vi "commandManipulateM1M3.vi"(8 "error in (no error)":errorcluster, 10 "CommandManipulateM1M3 in":T1, 11 "M1M3SAL in":refnum<class "M1M3SAL.lvclass">) -> (0 "error out":errorcluster, 2 "CommandManipulateM1M3 out":T1, 3 "M1M3SAL out":refnum<class "M1M3SAL.lvclass">)   [LabVIEW 2016, in "M1M3SupportCommunicator.lvlib" / "M1M3SAL.lvclass"]
uses:
  M1M3SAL.lvclass
  DataTypes/Topics/CommandManipulateM1M3.ctl
  DataTypes/Topics/Parts/CommandId.ctl
  DataTypes/MessageHeader.ctl
  DataTypes/MessageTypes.ctl
  DataTypes/MessageTopics.ctl
  M1M3SAL.lvclass/M1M3SAL.ctl
  writeU8.vi
  writeI32.vi
  M1M3SupportCommunicator.lvlib
  DataTypes/Topics/M1M3SupportTopics.lvlib
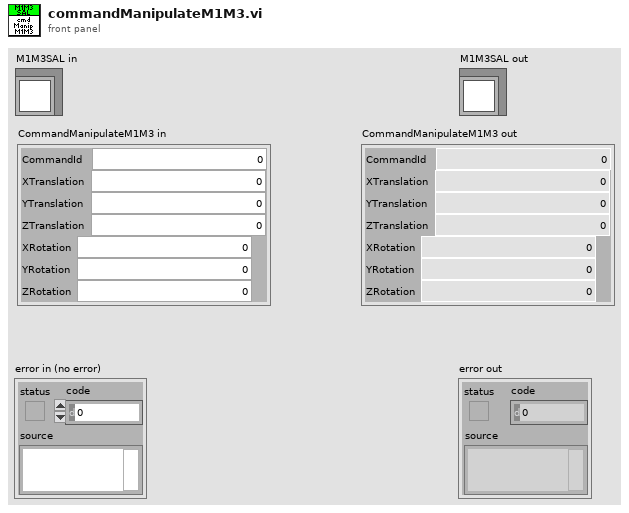
[diagram p1: front panel]
types:
  T1 = typedef "M1M3SupportTopics.lvlib/CommandManipulateM1M3.ctl" = cluster{"CommandId":T2, "XTranslation":dbl, "YTranslation":dbl, "ZTranslation":dbl, "XRotation":dbl, "YRotation":dbl, "ZRotation":dbl}
  T2 = typedef "M1M3SupportTopics.lvlib/CommandId.ctl" = i32
  T3 = typedef "M1M3SupportCommunicator.lvlib/MessageHeader.ctl" = cluster{"Type":T4, "Topic":T5, "Size":i32}
  T4 = typedef "M1M3SupportCommunicator.lvlib/MessageTypes.ctl" = enum8{"None", "PutSample", "GetNextSample", "LogEvent", "GetEvent", "IssueCommand", "CommandId", "WaitForCompletion", "AcceptCommand", "AckCommand"}
  T5 = typedef "M1M3SupportCommunicator.lvlib/MessageTopics.ctl" = enum8{"None", "ForceActuatorData", "MirrorForceData", "HardpointData", "AirData", "DynamicData", "FPGAData", "IMSData", "ForceActuatorStatus", "ElevationData", "HardpointStatus", "HardpointActuatorChase", "AirStatus", "ForceActuatorSafetyChecks", "ForceActuatorTest", "ActuatorBroadcastCounter", "StatusChecks", "CellChecks", "HardpointActuatorBreakaway", "RaiseMirrorComplete", "ILCCommunication", "ElevationAngleChecks", "DetailedState", "ServoLoops", "ForceActuatorInfo", "LowerMirrorComplete", "HardpointActuatorInfo", "SettingsApplied", "ErrorCode", "StartupChecks", "SummaryState", "SettingVersions", "ActuatorTestStatus", "AppliedSettingsMatchStart", "Enable", "EnterMaintenance", "Standby", "AbortLowerM1M3", "ApplyAberrationByForces", "ApplyAOSCorrectionByBendingModes", "ClearAOSCorrection", "Start", "RaiseM1M3", "TestForceActuator", "LowerM1M3", "ApplyAOSCorrectionByForces", "Disable", "ApplyAberationByBendingMode", "TestHardpoint", "ManipulateM1M3", "ClearAberration", "Exit", "TestAir", "AbortRaiseM1M3", "MoveHardpointActuators", "ExitMaintenance", "Shutdown"}
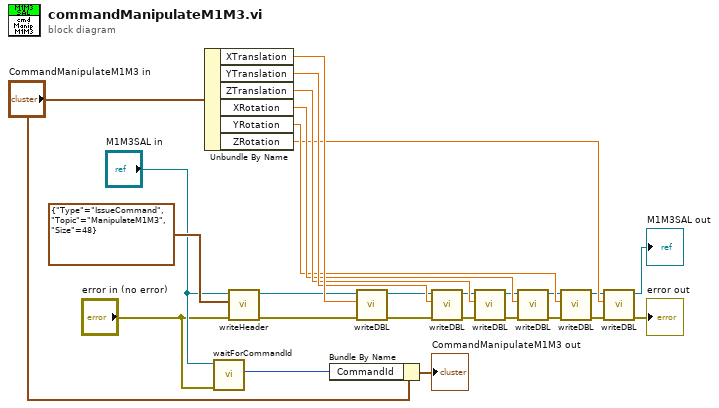
[diagram p0: block diagram]
diagram:
  n1 = Unbundle By Name("CommandManipulateM1M3 in") -> ("XTranslation"=w21:dbl, "YTranslation"=w20:dbl, "ZTranslation"=w19:dbl, "XRotation"=w18:dbl, "YRotation"=w17:dbl, "ZRotation"=w16:dbl)
  n2 = call "waitForCommandId.vi"("error in (no error)"="error in (no error)", "M1M3SAL in"="M1M3SAL in") -> ("CommandId"=w25:T2)  [unwired: 7 in, 2 out]
  n3 = call "writeHeader.vi"("error in (no error)"="error in (no error)", "MessageHeader"=T3 {"Type"=enum."IssueCommand", "Topic"=enum."ManipulateM1M3", "Size"=48}, "M1M3SAL in"="M1M3SAL in") -> ("error out"=w14:errorcluster, "M1M3SAL out"=w7:refnum<class "M1M3SAL.lvclass">)  [unwired: 7 in]
  n4 = Bundle By Name(cluster="CommandManipulateM1M3 in", "CommandId"=w25) -> (→"CommandManipulateM1M3 out":T1)
  n5 = call "writeDBL.vi"("error in (no error)"=w14, "Input"=w21, "M1M3SAL in"=w7) -> ("error out"=w13:errorcluster, "M1M3SAL out"=w6:refnum<class "M1M3SAL.lvclass">)  [unwired: 7 in]
  n6 = call "writeDBL.vi"("error in (no error)"=w13, "Input"=w20, "M1M3SAL in"=w6) -> ("error out"=w12:errorcluster, "M1M3SAL out"=w5:refnum<class "M1M3SAL.lvclass">)  [unwired: 7 in]
  n7 = call "writeDBL.vi"("error in (no error)"=w12, "Input"=w19, "M1M3SAL in"=w5) -> ("error out"=w11:errorcluster, "M1M3SAL out"=w4:refnum<class "M1M3SAL.lvclass">)  [unwired: 7 in]
  n8 = call "writeDBL.vi"("error in (no error)"=w11, "Input"=w18, "M1M3SAL in"=w4) -> ("error out"=w10:errorcluster, "M1M3SAL out"=w3:refnum<class "M1M3SAL.lvclass">)  [unwired: 7 in]
  n9 = call "writeDBL.vi"("error in (no error)"=w10, "Input"=w17, "M1M3SAL in"=w3) -> ("error out"=w9:errorcluster, "M1M3SAL out"=w2:refnum<class "M1M3SAL.lvclass">)  [unwired: 7 in]
  n10 = call "writeDBL.vi"("error in (no error)"=w9, "Input"=w16, "M1M3SAL in"=w2) -> ("error out"=→"error out":errorcluster, "M1M3SAL out"=→"M1M3SAL out":refnum<class "M1M3SAL.lvclass">)  [unwired: 7 in]
